vi "refreshNode.vi"(8 "error in (no error)":errorcluster, 10 "DataNode*":refnum<data-value>, 11 "xceRootNode in":refnum<class "xceRootNode.lvclass">) -> (0 "error out":errorcluster, 3 "xceRootNode out":refnum<class "xceRootNode.lvclass">)   [LabVIEW 2013, in "xceRootNode.lvclass"]
doc: "Refreshes a node in the tree control. Used when the name or text summary has potentially changed."
uses:
  xceRootNode.lvclass
  xceDataNode/xceDataNode.lvclass
  xceRootNode.lvclass/xceRootNode.ctl
  xceNode/xceNode.lvclass
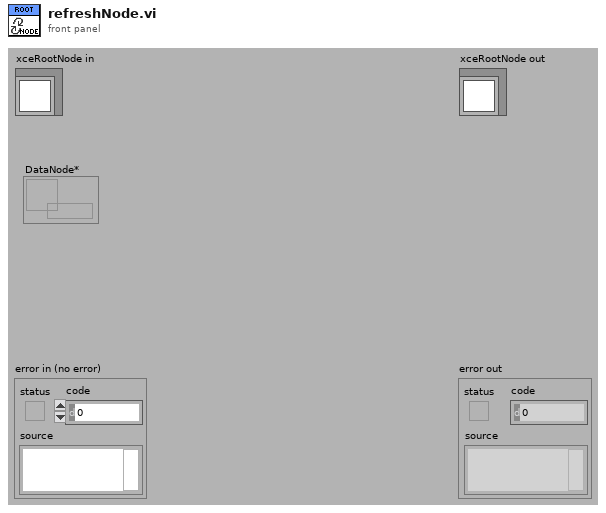
[diagram p1: front panel]
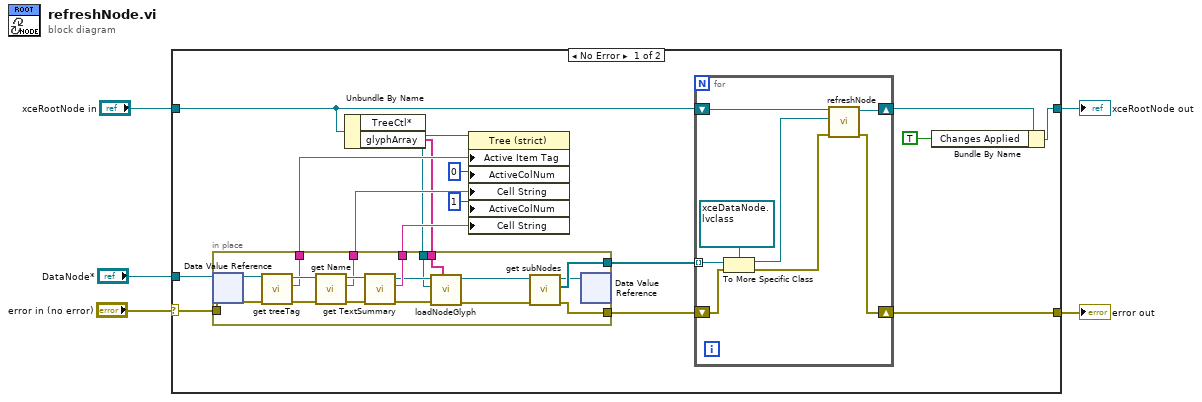
[diagram p0: block diagram]
diagram:
  n1 = case shown="No Error" "error in (no error)" {
    selector: "error in (no error)" -> [w18 w49]
    tunnel: [w11 w49] -> w4
    tunnel: [w8 w48] -> w2
    tunnel: "xceRootNode in" -> [w12 w48]
    tunnel: "DataNode*" -> [w21 _]
    frame No Error {
      n2 = Unbundle By Name(w12) -> ("TreeCtl*"=w7:refnum<vi>, "glyphArray"=w6:string[])
      n3 = in-place {
        in-place-border: w18 -> [w42]
        in-place-border: [w41] -> w17
        in-place-border: [w40] -> w16
        in-place-border: [w39] -> w15
        in-place-border: [w38] -> w13
        in-place-border: [w37] -> w14
        in-place-border: w7 -> [w31]
        in-place-border: w6 -> [w30]
        n4 = in-place-dvr #1(w21) -> (w47:refnum<class "xceDataNode.lvclass">)  [unwired: 1 out]
        n5 = call "get treeTag.vi"("error in (no error)"=w42, "xceNode in"=w47) -> ("error out"=w45:errorcluster, "treeTag"=w41:string, "xceNode out"=w46:refnum<class "xceDataNode.lvclass">)  [unwired: 7 in]
        n6 = call "get Name.vi"("error in (no error)"=w45, "xceDataNode in"=w46) -> ("error out"=w43:errorcluster, "Name"=w40:string, "xceDataNode out"=w44:refnum<class "xceDataNode.lvclass">)  [unwired: 7 in]
        n7 = call-dynamic "get TextSummary.vi"("error in (no error)"=w43, "xceDataNode in"=w44) -> ("error out"=w33:errorcluster, "Text Summary"=w39:string, "xceDataNode out"=w34:refnum<class "xceDataNode.lvclass">)  [unwired: 7 in]
        n8 = call "loadNodeGlyph.vi"("glyphArray"=w30, "error in (no error)"=w33, "TreeCtl* in"=w31, "xceDataNode in"=w34) -> ("error out"=w32:errorcluster, "xceDataNode out"=w35:refnum<class "xceDataNode.lvclass">)  [unwired: 5 in, 1 out]
        n9 = call "get subNodes.vi"("error in (no error)"=w32, "xceNode in"=w35) -> ("error out"=w38:errorcluster, "subNodes[]*"=w37:refnum<data-value>[], "xceNode out"=w36:refnum<class "xceDataNode.lvclass">)  [unwired: 7 in]
        n10 = in-place-dvr #1(w36) -> ()  [unwired: 2 out]
      }
      n11 = property class="Tree (strict)"(reference=w7, "Active Item Tag"=w17, "ActiveColNum"=0 ("Active Cell:Active Column Number"), "Cell String"=w16, "ActiveColNum"=1 ("Active Cell:Active Column Number"), "Cell String"=w15) -> ()  [unwired: 1 in, 2 out]
      n12 = for {
        tunnel: w14 -> [w29] mode=indexing
        shift-right: [w22] -> w11
        shift-left: w13 -> [w28]
        shift-right: [w24] -> w9
        shift-left: w12 -> [w25]
        n13 = To More Specific Class(target class=refnum<data-value> refnum ("DataNode*"), reference=w29, error in=w28) -> (specific class reference=w23:refnum<data-value>, error out=w26:errorcluster)
        n14 = call-dynamic "refreshNode.vi"("error in (no error)"=w26, "DataNode*"=w23, "xceRootNode in"=w25) -> ("error out"=w22:errorcluster, "xceRootNode out"=w24:refnum<class "xceRootNode.lvclass">)  [unwired: 7 in]
      }
      n15 = Bundle By Name(cluster=w9, "Changes Applied"=TRUE) -> (w8:refnum<class "xceRootNode.lvclass">)
    }
    frame Error {
    }
  }
  "error out" <- w4
  "xceRootNode out" <- w2
